vi "Lutron Parser.vi"(4 "ID":string) -> (2 "Control System":T1)   [LabVIEW 2016, in "Lutron QS Control Protocol.lvlib" / "Lutron QS Object.lvclass"]
uses:
  Lutron QS Object.lvclass
panel:
  out "Array - String":string[](array[string])
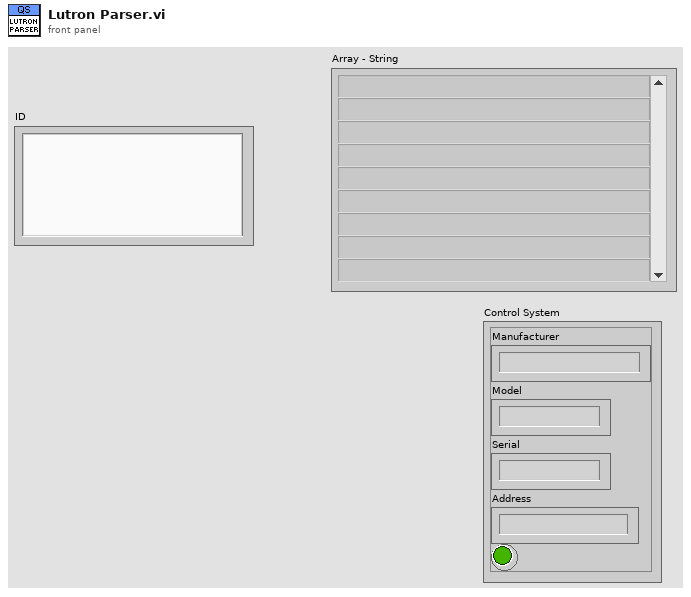
[diagram p1: front panel]
types:
  T1 = cluster{"Manufacturer":string, "Model":string, "Serial":string, "Address":string, "Boolean":bool}
  T2 = cluster{"Manufacturer":string, "Model":string, "Serial":string, "Address":string, bool}
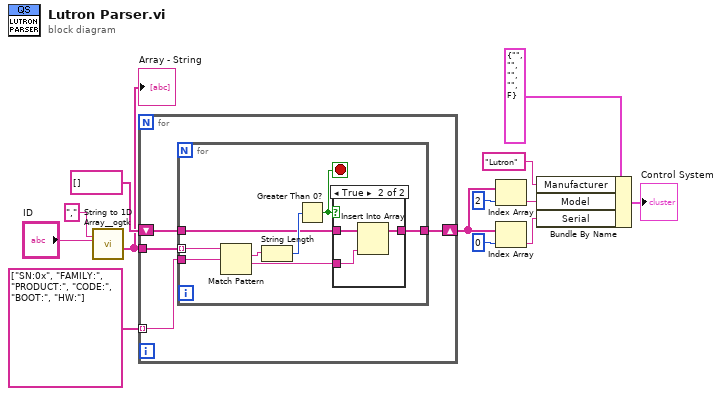
[diagram p0: block diagram]
diagram:
  n1 = call <userlib>:"String to 1D Array__ogtk.vi"("delimiter (Tab)"=",", "string"="ID") -> ("Array of Strings"=w12:string[])  [unwired: 9 in]
  "Array - String" <- w12
  n2 = for {
    tunnel: string[] ["SN:0x", "FAMILY:", "PRODUCT:", "CODE:", "BOOT:", "HW:"] -> [w16] mode=indexing
    tunnel: w12 -> [w17]
    shift-right: [w14] -> w5
    shift-left: string[] [] -> [w15]
    n3 = for {
      tunnel: w17 -> [w25] mode=indexing
      tunnel: w16 -> [w24]
      tunnel: w15 -> [w21]
      tunnel: [w19] -> w14
      stop <- w22 stop-if-true
      n4 = Match Pattern(string=w25, regular expression=w24) -> (match substring=w20:string, after substring=w18:string)  [unwired: 1 in, 2 out]
      n5 = String Length(string=w20) -> (length=w23:i32)
      n6 = Greater Than 0?(x=w23) -> (x > 0?=w22:bool)
      n7 = case shown="True" w22 {
        tunnel: w21 -> [w26 w29]
        tunnel: w18 -> [_ w28]
        tunnel: [w26 w27] -> w19
        frame False {
        }
        frame True {
          n8 = Insert Into Array(array=w29, new element=w28) -> (w27:string[])  [unwired: 1 in]
        }
      }
    }
  }
  n9 = Index Array(array=w5, index=2) -> (element=w6:string)
  n10 = Index Array(array=w5, index=0) -> (element=w4:string)
  n11 = Bundle By Name(cluster=T2 {"Manufacturer"="", "Model"="", "Serial"="", "Address"="", FALSE} ("Instrument"), "Manufacturer"="Lutron", "Model"=w6, "Serial"=w4) -> (→"Control System":T2)
